vi "ROI entry-ROI within img boundary-core.vi"(9 "Image resolution":i32, 10 "ROI Max (zero based)":i32, 11 "ROI Min (zero based)":i32) -> (2 "ROI Max":i32, 3 "ROI Min":i32)   [LabVIEW 2017]
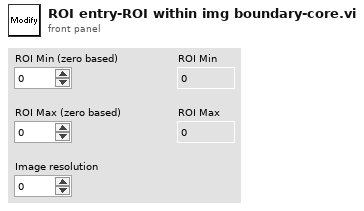
[diagram p1: front panel]
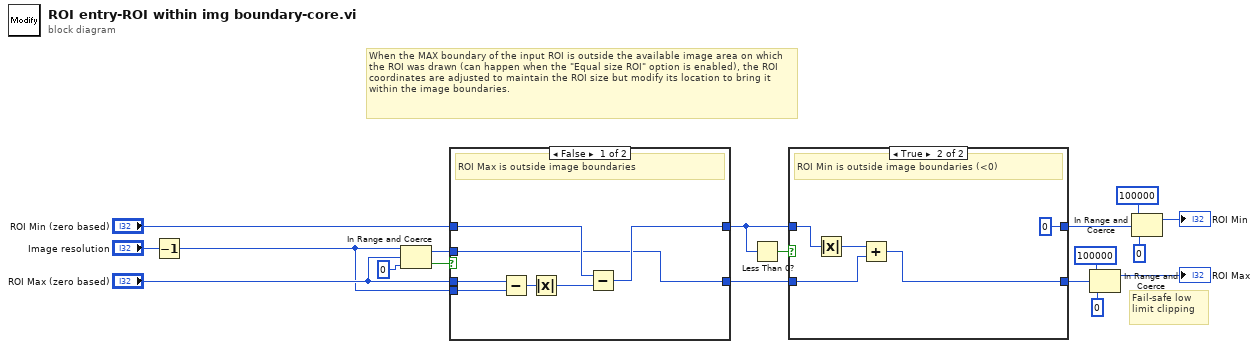
[diagram p0: block diagram]
diagram:
  # "When the MAX boundary of the input ROI is outside the available image area on which the ROI was drawn (can happen when the \"Equal size ROI\" option is enabled), the ROI coordinates are adjusted to maintain the ROI size but modify its location to bring it within the image boundaries."
  # "Fail-safe low limit clipping"
  n1 = Decrement(x="Image resolution") -> (x-1=w1:i32)
  n2 = In Range and Coerce(upper limit=w1, x="ROI Max (zero based)", lower limit=0) -> (coerced(x)=w7:i32, In Range?=w8:bool)
  n3 = case shown="False" w8 {
    tunnel: w7 -> [w19 _]
    tunnel: w1 -> [w23 _]
    tunnel: "ROI Min (zero based)" -> [w22 w27]
    tunnel: "ROI Max (zero based)" -> [w24 w26]
    tunnel: [w20 w27] -> w6
    tunnel: [w19 w26] -> w4
    frame False {
      # "ROI Max is outside image boundaries"
      n4 = Subtract(x=w24, y=w23) -> (x-y=w25:i32)
      n5 = Absolute Value(x=w25) -> (abs(x)=w21:i32)
      n6 = Subtract(x=w22, y=w21) -> (x-y=w20:i32)
    }
    frame True {
      # "ROI Max is within image boundaries"
    }
  }
  n7 = Less Than 0?(x=w6) -> (x < 0?=w2:bool)
  n8 = case shown="True" w2 {
    tunnel: w6 -> [w29 w34]
    tunnel: [w29 0 ("ROI Min")] -> w5
    tunnel: [w28 w30] -> w3
    tunnel: w4 -> [w28 w31]
    frame False {
      # "ROI Min is inside image boundaries (>0)"
    }
    frame True {
      # "ROI Min is outside image boundaries (<0)"
      n9 = Absolute Value(x=w34) -> (abs(x)=w32:i32)
      n10 = Add(x=w32, y=w31) -> (x+y=w30:i32)
    }
  }
  n11 = In Range and Coerce(upper limit=100000, x=w3, lower limit=0) -> (coerced(x)=→"ROI Max":i32)  [unwired: 1 out]
  n12 = In Range and Coerce(upper limit=100000, x=w5, lower limit=0) -> (coerced(x)=→"ROI Min":i32)  [unwired: 1 out]
